vi "databaseInset.vi"() -> ()   [LabVIEW 2024]
uses:
  <vilib>/addons/database/NI_Database_API.lvlib
  <vilib>/addons/database/Command.llb/Cmd Set Parameter Value (C).vi
  <vilib>/addons/database/Connection.llb/DB Tools Open Connec (String).vi
  <vilib>/addons/database/Command.llb/Cmd Delete.vi
  <vilib>/addons/database/Command.llb/Cmd Execute.vi
  <vilib>/addons/database/Recordset.llb/Rec Destroy - Command.vi
panel:
  in  "Parameterized SQL query":string="insert into inserttable (querytype, device, numsamples) values ('parameterized sql query', ?, ?) "
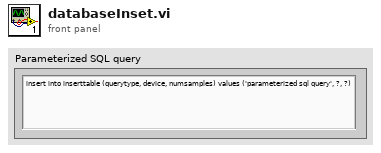
[diagram p1: front panel]
types:
  T1 = typedef "NI_Database_API.lvlib/Conn ObjectReference.ctl" = refnum<k1>
  T2 = typedef "NI_Database_API.lvlib/Cmd ObjectReference.ctl" = refnum<k1>
  T3 = typedef "NI_Database_API.lvlib/Cmd-Rec Object Reference.ctl" = refnum<k1>
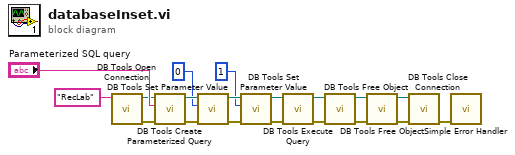
[diagram p0: block diagram]
diagram:
  n1 = call-poly <vilib>:"DB Tools Open Connection.vi"("connection information"="RecLab") -> ("error out"=w5:errorcluster, "connection reference"=w6:T1)  [unwired: 7 in]
  n2 = call <vilib>:"DB Tools Create Parameterized Query.vi"("error in (no error)"=w5, "SQL query"="Parameterized SQL query", "connection reference"=w6) -> ("error out"=w11:errorcluster, "command reference"=w14:T2)  [unwired: 4 in, 1 out]
  n3 = call-poly <vilib>:"DB Tools Set Parameter Value.vi"("error in (no error)"=w11, "parameter index"=0, "command reference"=w14) -> ("error out"=w13:errorcluster, "command reference out"=w12:T2)  [unwired: 5 in]
  n4 = call-poly <vilib>:"DB Tools Set Parameter Value.vi"("error in (no error)"=w13, "parameter index"=1, "command reference"=w12) -> ("error out"=w1:errorcluster, "command reference out"=w2:T2)  [unwired: 5 in]
  n5 = call-poly <vilib>:"DB Tools Execute Query.vi"("error in (no error)"=w1, "command reference"=w2) -> ("error out"=w15:errorcluster, "command-recordset reference"=w16:T3)  [unwired: 6 in]
  n6 = call-poly <vilib>:"DB Tools Free Object.vi"("error in (no error)"=w15, "command-recordset reference"=w16) -> ("error out"=w9:errorcluster, "command reference"=w17:T2)  [unwired: 8 in]
  n7 = call-poly <vilib>:"DB Tools Free Object.vi"("error in (no error)"=w9, "command reference"=w17) -> ("error out"=w3:errorcluster, "connection reference"=w4:T1)  [unwired: 8 in]
  n8 = call <vilib>:"DB Tools Close Connection.vi"("error in (no error)"=w3, "connection reference"=w4) -> ("error out"=w18:errorcluster)  [unwired: 5 in]
  n9 = call <vilib>:"Simple Error Handler.vi"("error in (no error)"=w18) -> ()  [unwired: 4 in, 5 out]
